vi "Write User Tag.vi"(8 "error in":errorcluster, 10 "user tag":i32, 11 "Has Timestamp in":refnum<class "Has Time Stamp.lvclass">) -> (0 "error out":errorcluster, 3 "Has Timestamp out":refnum<class "Has Time Stamp.lvclass">)   [LabVIEW 2020, in "PV Access.lvlib" / "PV Data.lvlib" / "Has Time Stamp.lvclass"]
uses:
  Has Time Stamp.lvclass
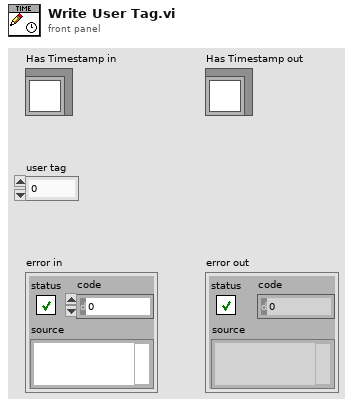
[diagram p1: front panel]
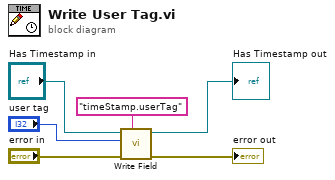
[diagram p0: block diagram]
diagram:
  n1 = call-dynamic "Write Field.vi"("field"="timeStamp.userTag" ("element name"), "error in (no error)"="error in", "value"="user tag", "Base Interface in"="Has Timestamp in") -> ("error out"=→"error out":errorcluster, "Base Interface out"=→"Has Timestamp out":refnum<class "Has Time Stamp.lvclass">)  [unwired: 6 in]
